vi "VISA to KNF Object.vi"(8 "error in (no error)":errorcluster, 11 "VISA resource name":refnum<visa-resource-name>) -> (0 "error out":errorcluster, 3 "SIMDOS out":refnum<class "SIMLAB_driver.lvclass">)   [LabVIEW 2018, in "KNF SIMDOS.lvlib"]
uses:
  KNF SIMDOS.lvlib
  <vilib>/KNF LAB/Driver S/Lvlib/SIMLAB_driver_lvclass/SIMLAB_driver.lvclass
  <vilib>/KNF LAB/Driver S/Lvlib/SIMLAB_driver_lvclass/InitParamCluster.ctl
  <vilib>/KNF LAB/Driver S/Lvlib/SIMLAB_driver_lvclass/PumpAddress.ctl
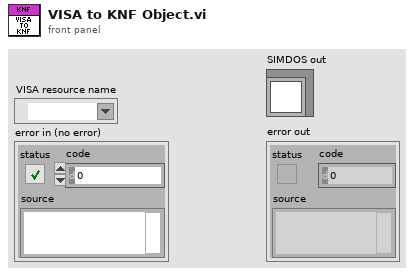
[diagram p1: front panel]
types:
  T1 = typedef "SIMLAB_driver.lvlib/SIMLAB_driver.lvclass/InitParamCluster.ctl" = cluster{"VISA resource name":refnum<visa-resource-name>, "Address":T2, "UnusedLRC":bool, "AckActive":bool}
  T2 = typedef "SIMLAB_driver.lvlib/SIMLAB_driver.lvclass/PumpAddress.ctl" = u8
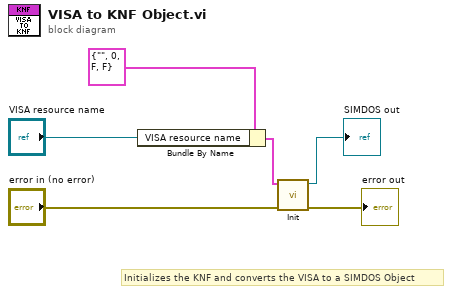
[diagram p0: block diagram]
diagram:
  # "Initializes the KNF and converts the VISA to a SIMDOS Object"
  n1 = Bundle By Name(cluster=T1 {"VISA resource name"="", "Address"=0, "UnusedLRC"=FALSE, "AckActive"=FALSE} ("InitParam"), "VISA resource name"="VISA resource name") -> (w5:T1)
  n2 = call <vilib>:"Init.vi"("error in (no error)"="error in (no error)", "InitParam"=w5) -> ("error out"=→"error out":errorcluster, "SIMDOS out"=→"SIMDOS out":refnum<class "SIMLAB_driver.lvclass">)  [unwired: 7 in, 1 out]
